vi "PCF8591-NX-DM.vi"(0 "Input of PCF8591-Nx":T1={"Compare High"=0, "Compare Low"=0, "Address"=144, "Vout"=255, "Control word"=64, "Set Vout"=FALSE} {"Control word" format="%x"; "Address" min=144 max=158 step=2 format="%x"; "Compare Low" format="%x"; "Compare High" format="%x"}, 2 "NXT":T2={"Hardware"="NXT", "Flattened String"=""}, 3 "Input Port":T3 items=["Port 1", "Port 2", "Port 3", "Port 4"]) -> (1 "Output of PCF8591-Nx":cluster{"Vin":u8, "Yes/No":bool}, 4 "NXT dup":T2={"Hardware"="NXT", "Flattened String"=""})   [LabVIEW 2010]
uses:
  <vilib>/NXT/Block Support/NXT_InputPort.ctl
  <vilib>/NXT/Subs/LVHSConnector.ctl
  <vilib>/NXT/Block Support/HWPage.SensorType.ctl
  <vilib>/NXT/Block Support/HWPage.SensorMode.ctl
panel:
  # "mindsensors.com\nCopyright (c) 2009 by mindsensors.com\nEmail: info (<at>) mindsensors (<dot>) com\n\nThis program is free software. You can redistribute it and/or modify\nit under the terms of the GNU General Public License as published by\nthe Free Software Foundation; version 3 of the License.\nRead the license at: http://www.gnu.org/licenses/gpl.txt"
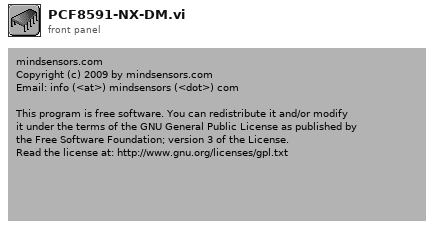
[diagram p1: front panel]
types:
  T1 = cluster{"Compare High":u8, "Compare Low":u8, "Address":u8, "Vout":u8, "Control word":u8, "Set Vout":bool}
  T2 = typedef "LVHSConnector.ctl" = cluster{"Hardware":string, "Flattened String":string}
  T3 = typedef "NXT_InputPort.ctl" = u8
  T4 = typedef "HWPage.SensorType.ctl" = u8
  T5 = typedef "HWPage.SensorMode.ctl" = u8
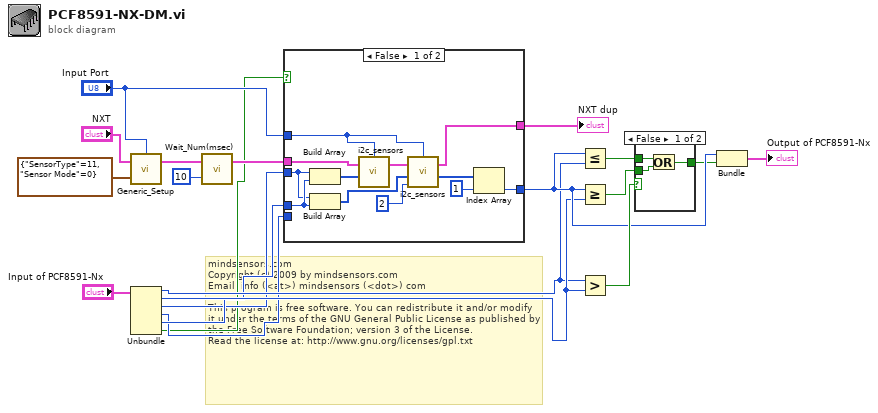
[diagram p0: block diagram]
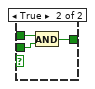
[diagram p2: hidden frame]
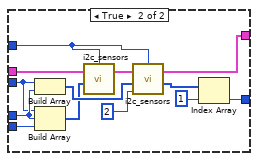
[diagram p3: hidden frame]
diagram:
  # "mindsensors.com\nCopyright (c) 2009 by mindsensors.com\nEmail: info (<at>) mindsensors (<dot>) com\n\nThis program is free software. You can redistribute it and/or modify\nit under the terms of the GNU General Public License as published by\nthe Free Software Foundation; version 3 of the License.\nRead the license at: http://www.gnu.org/licenses/gpl.txt"
  n1 = call <vilib>:"Generic_Setup.vi"("Sensor Setup"=cluster{"SensorType":T4, "Sensor Mode":T5} {"SensorType"=11, "Sensor Mode"=0}, "NXT"="NXT", "Port"="Input Port") -> ("NXT"=w14:T2)  [unwired: 1 out]
  n2 = Unbundle("Input of PCF8591-Nx") -> ("Compare High"=w5:u8, "Compare Low"=w6:u8, "Address"=w3:u8, "Vout"=w2:u8, "Control word"=w4:u8, "Set Vout"=w1:bool)
  n3 = call <vilib>:"Wait_Num(msec).vi"("Time (100 msec)"=u32 10 ("Time msec)"), "NXT"=w14) -> ("NXT"=w12:T2)  [unwired: 2 in]
  n4 = case shown="False" w1 {
    tunnel: w3 -> [w25 w34]
    tunnel: w2 -> [_ w45]
    tunnel: [w32 w44] -> w10
    tunnel: w4 -> [w27 w41]
    tunnel: "Input Port" -> [w29 w40]
    tunnel: w12 -> [w21 w39]
    tunnel: [w22 w37] -> w11
    frame False {
      n5 = Build Array(w25, w27) -> (w24:u8[])
      n6 = Build Array(w25, w27) -> (w28:u8[])
      n7 = call <vilib>:"i2c_sensors.vi"("Bytes to Write"=w24, "NXT"=w21, "Port"=w29) -> ("NXT"=w23:T2)  [unwired: 2 in, 2 out]
      n8 = call <vilib>:"i2c_sensors.vi"("Return Length"=u8 2 ("ReturnLength"), "Bytes to Write"=w28, "NXT"=w23, "Port"=w29) -> ("Bytes read"=w26:u8[], "NXT"=w22:T2)  [unwired: 1 in, 1 out]
      n9 = Index Array(array=w26, index=u8 1 ("register")) -> (element=w32:u8)
    }
    frame True {
      n10 = Build Array(w34, w41) -> (w42:u8[])
      n11 = Build Array(w34, w41, w45) -> (w33:u8[])
      n12 = call <vilib>:"i2c_sensors.vi"("Bytes to Write"=w33, "NXT"=w39, "Port"=w40) -> ("NXT"=w38:T2)  [unwired: 2 in, 2 out]
      n13 = call <vilib>:"i2c_sensors.vi"("Return Length"=u8 2 ("ReturnLength"), "Bytes to Write"=w42, "NXT"=w38, "Port"=w40) -> ("Bytes read"=w36:u8[], "NXT"=w37:T2)  [unwired: 1 in, 1 out]
      n14 = Index Array(array=w36, index=u8 1 ("register")) -> (element=w44:u8)
    }
  }
  "NXT dup" <- w11
  n15 = Less Or Equal?(x=w10, y=w5) -> (x <= y?=w18:bool)
  n16 = Greater Or Equal?(x=w10, y=w6) -> (x >= y?=w19:bool)
  n17 = Greater?(x=w5, y=w6) -> (0:w20:bool)
  n18 = case shown="False" w20 {
    tunnel: [w46 w51] -> w9
    tunnel: w18 -> [w48 w50]
    tunnel: w19 -> [w47 w49]
    frame False {
      n19 = Or(x=w48, y=w47) -> (x .or. y?=w46:bool)
    }
    frame True {
      n20 = And(x=w50, y=w49) -> (x .and. y?=w51:bool)
    }
  }
  n21 = Bundle(w10, w9) -> (→"Output of PCF8591-Nx":cluster{u8, bool})  [unwired: 1 in]
